vi "sync.vi"(8 "error in (no error)":errorcluster, 11 "5785_3.2GHz_one channel in":refnum<class "5785_3.2GHz_one channel.lvclass">) -> (0 "error out":errorcluster, 3 "5785_3.2GHz_one channel out":refnum<class "5785_3.2GHz_one channel.lvclass">)   [LabVIEW 2021, in "5785_3.2GHz_one channel.lvclass"]
uses:
  5785_3.2GHz_one channel.lvclass
  5785_3.2GHz_one channel.lvclass/5785_3.2GHz_one channel.ctl
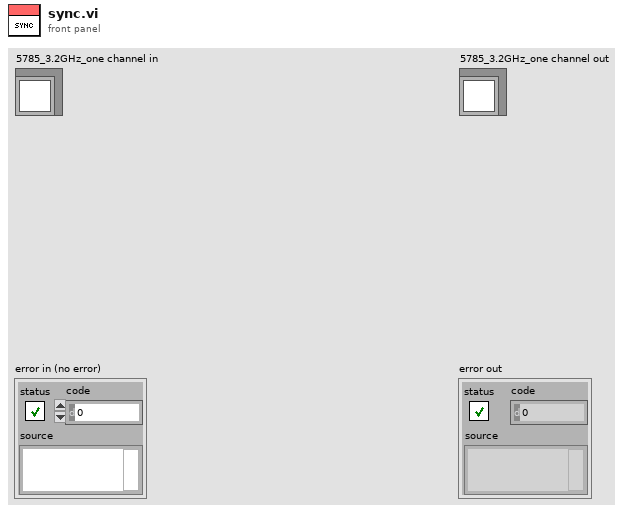
[diagram p1: front panel]
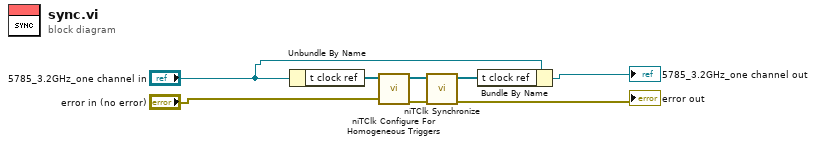
[diagram p0: block diagram]
diagram:
  n1 = Unbundle By Name("5785_3.2GHz_one channel in") -> ("t clock ref"=w6:refnum<k20>[])
  n2 = call <instrlib>:"niTClk Configure For Homogeneous Triggers.vi"("error in (no error)"="error in (no error)", "sessions"=w6) -> ("error out"=w7:errorcluster, "sessions out"=w8:refnum<k20>[])  [unwired: 8 in]
  n3 = call <instrlib>:"niTClk Synchronize.vi"("error in (no error)"=w7, "sessions"=w8) -> ("error out"=→"error out":errorcluster, "sessions out"=w5:refnum<k20>[])  [unwired: 8 in]
  n4 = Bundle By Name(cluster="5785_3.2GHz_one channel in", "t clock ref"=w5) -> (→"5785_3.2GHz_one channel out":refnum<class "5785_3.2GHz_one channel.lvclass">)
